vi "Configure Math (Basic).vi"(6 "Operator (0:Add)":u16(ring) items=["Add", "Subtract", "Multiply", "Divide"], 7 "Destination (4:Math1)":u16(ring)=4 items=["Math1"=4, "Math2"=5, "Math3"=6, "Math4"=7], 8 "error in (no error)":errorcluster, 9 "Source 2 (1:Channel2)":u16(ring)=1 items=["Channel1", "Channel2", "Channel3", "Channel4", "Math1", "Math2", "Math3", "Math4", "Reference1", "Reference2", "Reference3", "Reference4"], 10 "Source 1 (0:Channel1)":u16(ring) items=["Channel1", "Channel2", "Channel3", "Channel4", "Math1", "Math2", "Math3", "Math4", "Reference1", "Reference2", "Reference3", "Reference4"], 11 "VISA resource name":refnum<visa-resource-name>) -> (0 "error out":errorcluster, 3 "VISA resource name out":refnum<visa-resource-name>)   [LabVIEW 2011, in "Tektronix 7000 Series.lvlib"]
doc: "Configures a math channel for standard waveform math operations such as add, subtract, multiply, and divide."
uses:
  Tektronix 7000 Series.lvlib
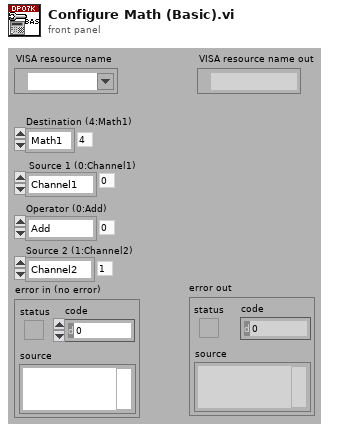
[diagram p1: front panel]
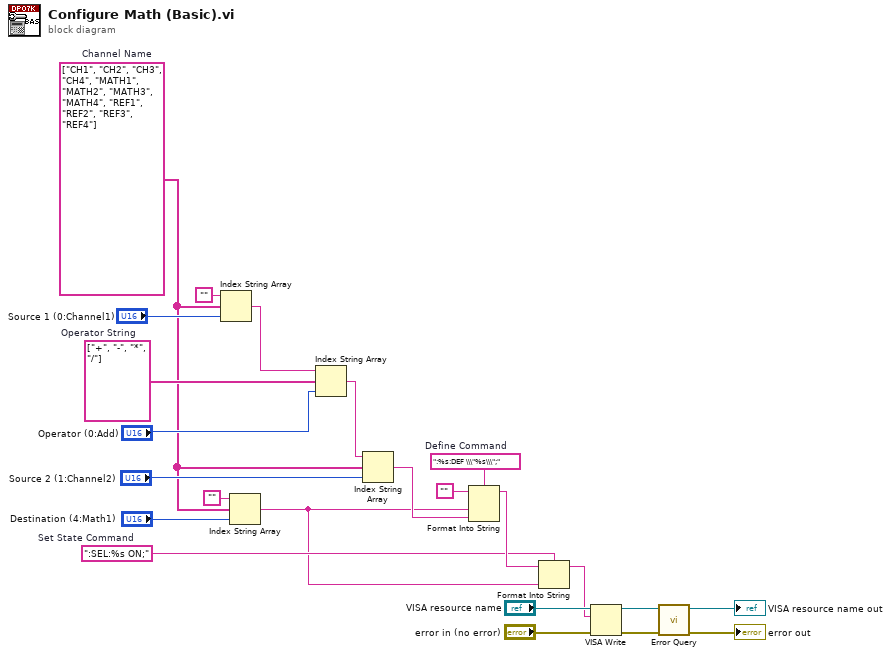
[diagram p0: block diagram]
diagram:
  w5 = ":SEL:%s ON;"  # Set State Command
  w7 = string[] ["CH1", "CH2", "CH3", "CH4", "MATH1", "MATH2", "MATH3", "MATH4", "REF1", "REF2", "REF3", "REF4"]  # Channel Name
  w16 = ":%s:DEF \\\"%s\\\";"  # Define Command
  w21 = string[] ["+", "-", "*", "/"]  # Operator String
  n1 = Index String Array(1:"Source 1 (0:Channel1)", 2:w7, 3:"") -> (0:w23:string)
  n2 = Index String Array(1:"Destination (4:Math1)", 2:w7, 3:"") -> (0:w4:string)
  n3 = Index String Array(1:"Operator (0:Add)", 2:w21, 3:w23) -> (0:w22:string)
  n4 = Index String Array(1:"Source 2 (1:Channel2)", 2:w7, 3:w22) -> (0:w12:string)
  n5 = Format Into String(format string=w16, initial string="", w4, w12) -> (resulting string=w6:string)  [unwired: 1 in, 1 out]
  n6 = Format Into String(format string=w5, initial string=w6, w4) -> (resulting string=w3:string)  [unwired: 1 in, 1 out]
  n7 = VISA Write(VISA resource name="VISA resource name", write buffer=w3, error in (no error)="error in (no error)") -> (VISA resource name out=w11:refnum<visa-resource-name>, error out=w10:errorcluster)  [unwired: 1 out]
  n8 = call "Error Query.vi"("error in (no error)"=w10, "VISA resource name"=w11) -> ("error out"=→"error out":errorcluster, "VISA resource name out"=→"VISA resource name out":refnum<visa-resource-name>)  [unwired: 6 in, 2 out]
